vi "ADC GOBLIN2.vi"() -> ()   [LabVIEW 2014]
uses:
  <vilib>/Instr/_visa.llb/VISA Configure Serial Port (Instr).vi
panel:
  out "?":i32(graph)
  out "ADC GOBLIN 2":dbl(slide) scale=0.0..1024.0
  in  "?":refnum<visa-resource-name>
  out "HIGH":bool
  out "MEDIUM":bool
  out "LOW":bool
  out "BITS":dbl
  in  "?":bool
  # "COM"
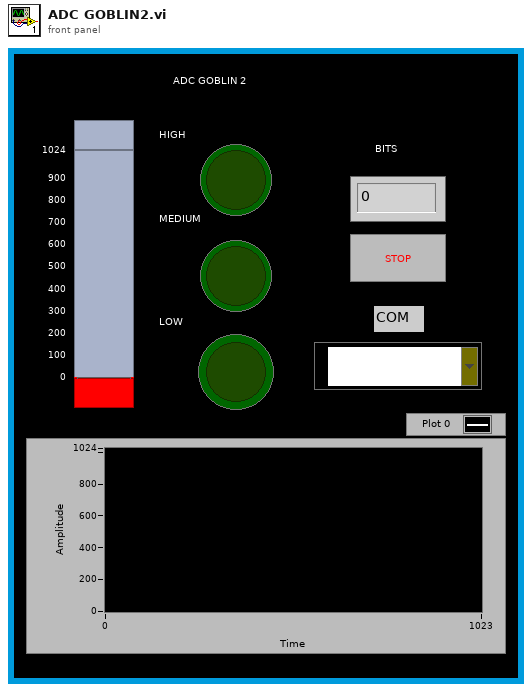
[diagram p1: front panel]
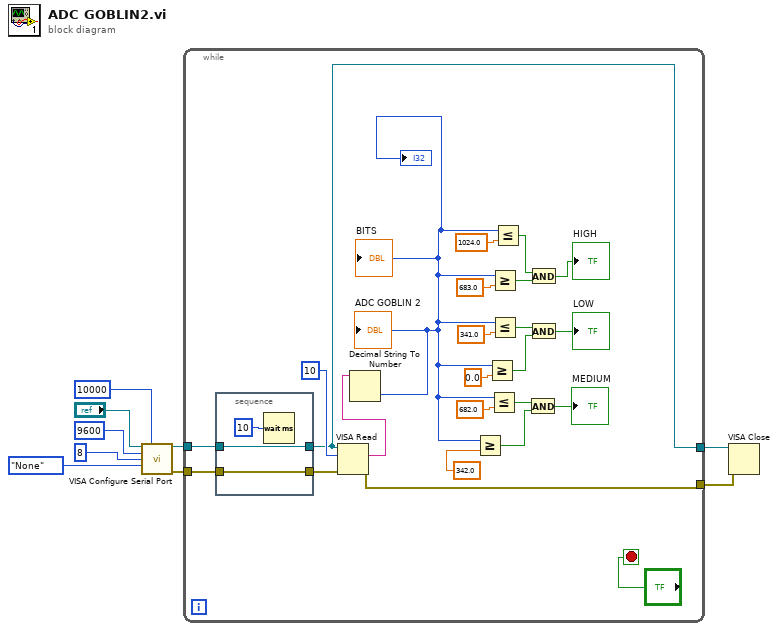
[diagram p0: block diagram]
diagram:
  n1 = call-poly "VISA Configure Serial Port"("VISA resource name"="?", "timeout (10sec)"=u32 10000, "baud rate (9600)"=u32 9600, "data bits (8)"=u16 8, "parity (0:none)"=enum16{"None", "Odd", "Even", "Mark", "Space"}."None") -> ("VISA resource name out"=w4:refnum<visa-resource-name>, "error out"=w3:errorcluster)  [unwired: 9 in]
  n2 = while {
    tunnel: w3 -> [w15]
    tunnel: w4 -> [w14]
    tunnel: [w12] -> w2
    tunnel: [w13] -> w1
    stop <- "?" stop-if-true
    n3 = stacked-sequence {
      tunnel: [w36] -> w12
      tunnel: w14 -> [w36]
      tunnel: [w35] -> w17
      tunnel: w15 -> [w35]
      frame #0 {
        n4 = Wait (ms)(milliseconds to wait=u32 10) -> ()  [unwired: 1 out]
      }
    }
    n5 = VISA Read(VISA resource name=w12, byte count=u32 10, error in (no error)=w17) -> (read buffer=w11:string, error out=w13:errorcluster)  [unwired: 2 out]
    n6 = Decimal String To Number(string=w11) -> (number=w10:i32)  [unwired: 2 in, 1 out]
    "BITS" <- w10
    "ADC GOBLIN 2" <- w10
    "?" <- w10
    n7 = Greater Or Equal?(x=w10, y=342.0) -> (x >= y?=w24:bool)
    n8 = Greater Or Equal?(x=w10, y=0.0) -> (x >= y?=w28:bool)
    n9 = Less Or Equal?(x=w10, y=682.0) -> (x <= y?=w25:bool)
    n10 = Greater Or Equal?(x=w10, y=683.0) -> (x >= y?=w19:bool)
    n11 = Less Or Equal?(x=w10, y=341.0) -> (x <= y?=w29:bool)
    n12 = Less Or Equal?(x=w10, y=1024.0) -> (x <= y?=w20:bool)
    n13 = And(x=w25, y=w24) -> (x .and. y?=→"MEDIUM":bool)
    n14 = And(x=w20, y=w19) -> (x .and. y?=→"HIGH":bool)
    n15 = And(x=w29, y=w28) -> (x .and. y?=→"LOW":bool)
  }
  n16 = VISA Close(VISA resource name=w2, error in (no error)=w1) -> ()  [unwired: 1 out]
